vi "Wait For Homed.vi"(8 "error in (no error)":errorcluster, 10 "Process State":refnum<data-value>, 11 "iMotion Controller in":refnum<class "iMotion Controller.lvclass">) -> (0 "error out":errorcluster)   [LabVIEW 2022 SP3, in "XY Stage Process.lvlib" / "XY Stage Process.lvclass"]
uses:
  XY Stage Process.lvclass
  Axis Objects/iMotion Controller/iMotion Controller.lvclass
  Process State Data/Process State Data.lvclass
  Process State Data/Process State Data.lvclass/Process State Data.ctl
  Process State Data/Accessor/Read Abort.vi
  XY Stage Process.lvclass/XY Stage Process.ctl
  <vilib>/ErrorRing/Error Ring.xnode
  <vilib>/Utility/error.llb/Error Cluster From Error Code.vi
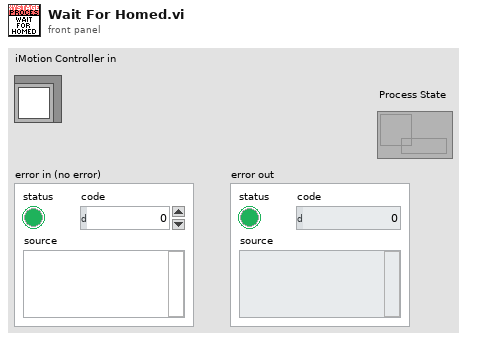
[diagram p1: front panel]
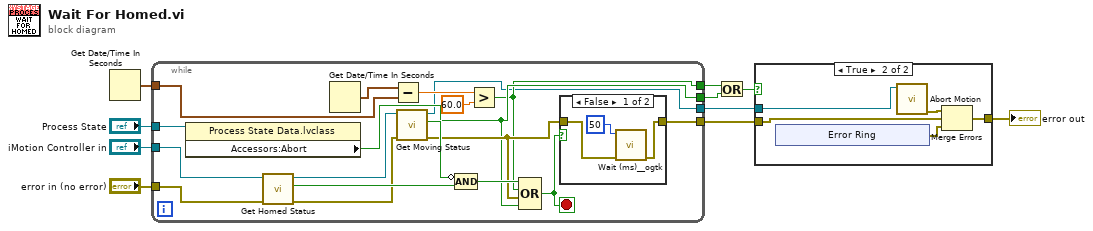
[diagram p0: block diagram]
diagram:
  n1 = Get Date/Time In Seconds() -> (seconds since 1Jan1904=w8:timestamp)
  n2 = while {
    tunnel: "error in (no error)" -> [w18]
    tunnel: [w23] -> w2
    tunnel: w8 -> [w26]
    tunnel: "iMotion Controller in" -> [w17]
    tunnel: "Process State" -> [w14]
    tunnel: [w13] -> w6
    tunnel: [w12] -> w5
    tunnel: [w11] -> w3
    stop <- w22 stop-if-true
    n3 = property class="Process State Data.lvclass"(reference=w14) -> ("Accessors:Abort"=w13:bool)  [unwired: 1 in, 2 out]
    n4 = call-dynamic "Get Homed Status.vi"("error in (no error)"=w18, "iMotion Controller in"=w17) -> ("error out"=w15:errorcluster, "Homed"=w19:bool, "iMotion Controller out"=w16:refnum<class "iMotion Controller.lvclass">)  [unwired: 7 in]
    n5 = Get Date/Time In Seconds() -> (seconds since 1Jan1904=w27:timestamp)
    n6 = Subtract(x=w27, y=w26) -> (x-y=w24:dbl)
    n7 = call-dynamic "Get Moving Status.vi"("error in (no error)"=w15, "iMotion Controller in"=w16) -> ("error out"=w20:errorcluster, "Moving"=w21:bool, "iMotion Controller out"=w11:refnum<class "iMotion Controller.lvclass">)  [unwired: 7 in]
    n8 = Compound Arithmetic op=AND(invert w21, w19) -> (w28:bool)
    n9 = Greater?(x=w24, y=60.0 ("x")) -> (0:w12:bool)
    n10 = Compound Arithmetic op=OR(w28, w12, w20, w13) -> (w22:bool)
    n11 = case shown="False" w22 {
      tunnel: w20 -> [w31 w32]
      tunnel: [w30 w32] -> w23
      frame False {
        n12 = call <userlib>:"Wait (ms)__ogtk.vi"("error in (no error)"=w31, "milliseconds to wait"=u32 50) -> ("error out"=w30:errorcluster)  [unwired: 8 in, 1 out]
      }
      frame True {
      }
    }
  }
  n13 = Or(x=w5, y=w6) -> (x .or. y?=w4:bool)
  n14 = case shown="True" w4 {
    tunnel: w3 -> [_ w38]
    tunnel: w2 -> [w33 w35]
    tunnel: [w33 w36] -> w1
    frame False {
    }
    frame True {
      n15 = xnode "Error Ring"() -> ("error out"=w34:errorcluster)
      n16 = call-dynamic "Abort Motion.vi"("iMotion Controller in"=w38) -> ("error out"=w37:errorcluster)  [unwired: 9 in, 1 out]
      n17 = Merge Errors(w37, w35, w34) -> (w36:errorcluster)
    }
  }
  "error out" <- w1
